vi "ClusterToValueList.vi"(9 "Name prefix":string, 10 "ValueList (empty)":cluster{"Label":string, "Value":string}[](array[cluster]), 11 "Cluster Refnum":refnum<vi>) -> (3 "ValueList (out)":cluster{"Label":string, "Value":string}[](array[cluster]))   [LabVIEW 2011]
panel:
  out "Array 2":variant[](array[variant])
  out "Array":string[](array[string])
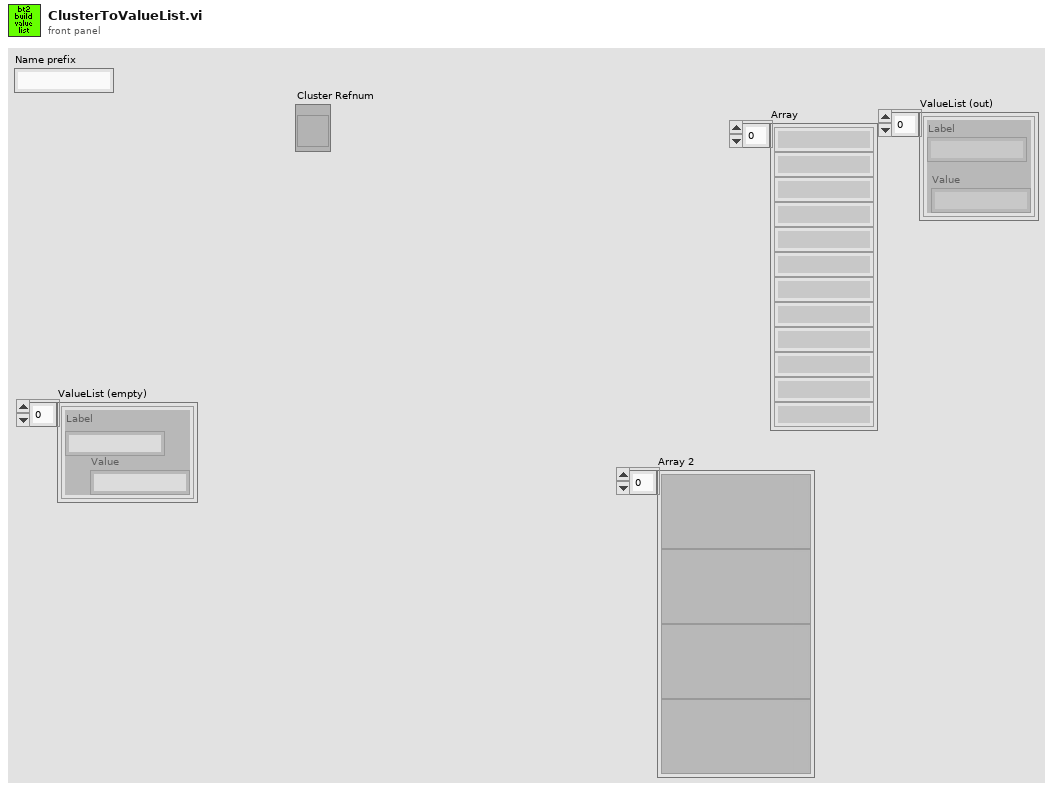
[diagram p1: front panel]
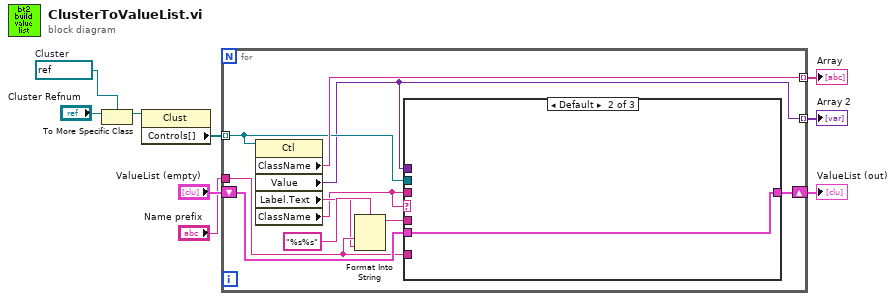
[diagram p0: block diagram]
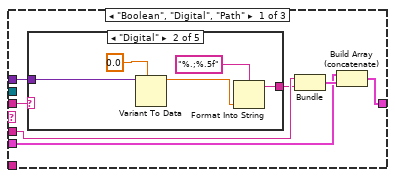
[diagram p2: hidden frame]
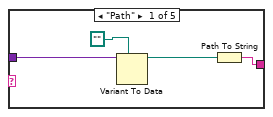
[diagram p3: hidden frame]
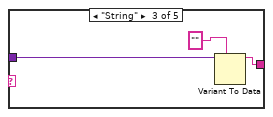
[diagram p4: hidden frame]
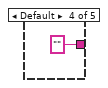
[diagram p5: hidden frame]
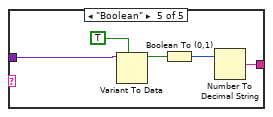
[diagram p6: hidden frame]
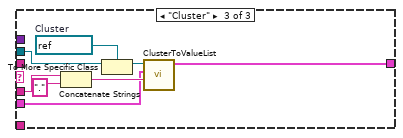
[diagram p7: hidden frame]
diagram:
  w2 = refnum<vi> refnum  # Cluster
  n1 = To More Specific Class(target class=w2, reference="Cluster Refnum") -> (specific class reference=w3:refnum<vi>)  [unwired: 1 in, 1 out]
  n2 = property class="Clust"(reference=w3) -> ("Controls[]"=w9:refnum<vi>[])  [unwired: 1 in, 2 out]
  n3 = for {
    tunnel: w9 -> [w18] mode=indexing
    tunnel: [w19] -> w8 mode=indexing
    tunnel: [w15] -> w7 mode=indexing
    shift-right: [w17] -> w1
    shift-left: "ValueList (empty)" -> [w16]
    tunnel: "Name prefix" -> [w13]
    n4 = property class="Ctl"(reference=w18) -> ("ClassName"=w19:string, "Value"=w15:variant, "Label.Text"=w12:string, "ClassName"=w10:string)  [unwired: 1 in, 2 out]
    n5 = Format Into String(format string="%s%s", w13, w12) -> (resulting string=w11:string)  [unwired: 2 in, 1 out]
    n6 = case shown="Default" w10 {
      tunnel: w18 -> [_ _ w53]
      tunnel: w16 -> [w22 w45 w46]
      tunnel: [w21 w45 w50] -> w17
      tunnel: w13 -> [_ _ _]
      tunnel: w15 -> [w20 _ _]
      tunnel: w11 -> [w25 _ w49]
      tunnel: w10 -> [w24 _ _]
      frame "Boolean", "Digital", "Path" {
        n7 = case shown="\"Digital\"" w24 {
          tunnel: [w27 w33 w36 "" w40] -> w23
          tunnel: w20 -> [w29 w35 w37 _ w43]
          frame "Path" {
            n8 = Variant To Data(type=path "", Variant=w29) -> (data=w28:path)  [unwired: 1 in, 1 out]
            n9 = Path To String(path=w28) -> (string=w27:string)
          }
          frame "Digital" {
            n10 = Variant To Data(type=0.0, Variant=w35) -> (data=w32:dbl)  [unwired: 1 in, 1 out]
            n11 = Format Into String(format string="%.;%.5f", w32) -> (resulting string=w33:string)  [unwired: 2 in, 1 out]
          }
          frame "String" {
            n12 = Variant To Data(type="", Variant=w37) -> (data=w36:string)  [unwired: 1 in, 1 out]
          }
          frame Default {
          }
          frame "Boolean" {
            n13 = Variant To Data(type=TRUE, Variant=w43) -> (data=w42:bool)  [unwired: 1 in, 1 out]
            n14 = Boolean To (0,1)(Boolean=w42) -> (0, 1=w41:i16)
            n15 = Number To Decimal String(number=w41) -> (decimal integer string=w40:string)  [unwired: 1 in]
          }
        }
        n16 = Bundle(w25, w23) -> (w26:cluster{string, string})  [unwired: 1 in]
        n17 = Build Array (concatenate)(w22, w26) -> (w21:cluster{"Label":string, "Value":string}[])
      }
      frame Default {
      }
      frame "Cluster" {
        w52 = refnum<vi> refnum  # Cluster
        n18 = Concatenate Strings(w49, "." ("string")) -> (w47:string)
        n19 = To More Specific Class(target class=w52, reference=w53) -> (specific class reference=w51:refnum<vi>)  [unwired: 1 in, 1 out]
        n20 = call "ClusterToValueList.vi"("Name prefix"=w47, "ValueList (empty)"=w46, "Cluster Refnum"=w51) -> ("ValueList (out)"=w50:cluster{"Label":string, "Value":string}[])  [unwired: 8 in]
      }
    }
  }
  "Array" <- w8
  "Array 2" <- w7
  "ValueList (out)" <- w1
